vi "getClockInfo.vi"(8 "error in (no error)":errorcluster, 11 "DeviceData in":refnum<class "DeviceData.lvclass">) -> (0 "error out":errorcluster, 1 "masterClockRate":dbl, 2 "clock":string, 3 "DeviceData out":refnum<class "DeviceData.lvclass">, 4 "start_trigger":string)   [LabVIEW 2011, in "DataMappers.lvlib" / "DeviceData.lvclass"]
uses:
  DeviceData.lvclass
  DeviceData.lvclass/DeviceData.ctl
  DatabaseHelpers/Database Objects/device/device.lvclass
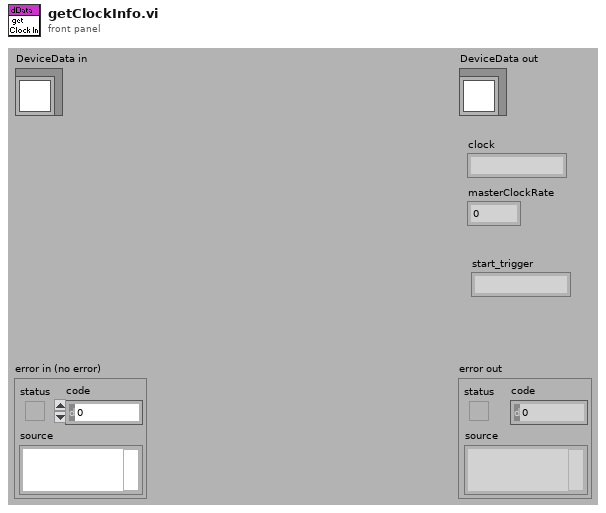
[diagram p1: front panel]
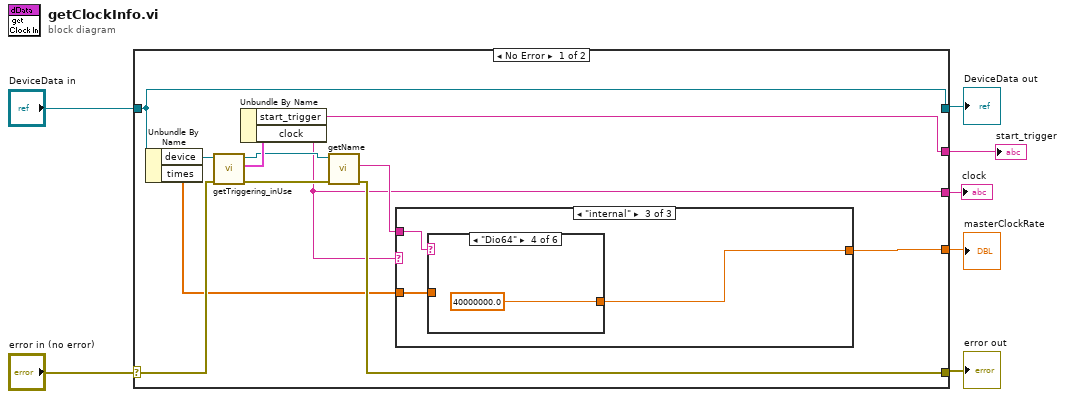
[diagram p0: block diagram]
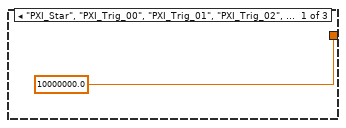
[diagram p2: hidden frame]
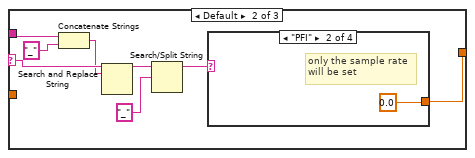
[diagram p3: hidden frame]
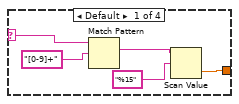
[diagram p4: hidden frame]
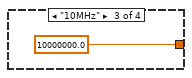
[diagram p5: hidden frame]
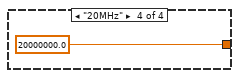
[diagram p6: hidden frame]
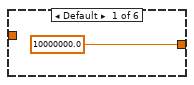
[diagram p7: hidden frame]
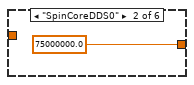
[diagram p8: hidden frame]
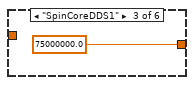
[diagram p9: hidden frame]
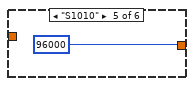
[diagram p10: hidden frame]
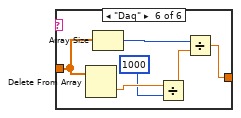
[diagram p11: hidden frame]
diagram:
  n1 = case shown="No Error" "error in (no error)" {
    selector: "error in (no error)" -> [w17 w52]
    tunnel: [w12 w52] -> w6
    tunnel: [w19 w51] -> w4
    tunnel: "DeviceData in" -> [w19 w51]
    tunnel: [w11 _] -> w3
    tunnel: [w10 _] -> w2
    tunnel: [w9 _] -> w1
    frame No Error {
      n2 = Unbundle By Name(w19) -> ("device"=w18:refnum<class "device.lvclass">, "times"=w8:dbl[])
      n3 = call "getTriggering_inUse.vi"("error in (no error)"=w17, "device.lvclass in"=w18) -> ("error out"=w14:errorcluster, "triggering_inUse"=w16:cluster{"start_trigger":string, "clock":string}, "device.lvclass out"=w15:refnum<class "device.lvclass">)  [unwired: 7 in]
      n4 = Unbundle By Name(w16) -> ("start_trigger"=w9:string, "clock"=w11:string)
      n5 = call "getName.vi"("error in (no error)"=w14, "device.lvclass in"=w15) -> ("error out"=w12:errorcluster, "name"=w13:string)  [unwired: 7 in, 1 out]
      n6 = case shown="\"internal\"" w11 {
        selector: w11 -> [_ w26 _]
        tunnel: w13 -> [_ w28 w39]
        tunnel: [10000000.0 w24 w38] -> w10
        tunnel: w8 -> [_ _ w37]
        frame "PXI_Star", "PXI_Trig_00", "PXI_Trig_01", "PXI_Trig_02", "PXI_Trig_03", "PXI_Trig_04", "PXI_Trig_05", "PXI_Trig_06", "PXI_Trig_07" {
        }
        frame Default {
          n7 = Concatenate Strings(w28, "_") -> (w25:string)
          n8 = Search and Replace String(input string=w26, search string=w25) -> (result string=w23:string)  [unwired: 6 in, 3 out]
          n9 = Search/Split String(string=w23, search string/char (-)="_") -> (substring before match=w21:string)  [unwired: 1 in, 2 out]
          n10 = case shown="\"PFI\"" w21 {
            selector: w21 -> [w33 _ _ _]
            tunnel: [w31 0.0 10000000.0 20000000.0] -> w24
            frame Default {
              n11 = Match Pattern(string=w33, regular expression="[0-9]+") -> (match substring=w30:string)  [unwired: 1 in, 3 out]
              n12 = Scan Value(string=w30, format string="%15") -> (value=w31:dbl)  [unwired: 1 in, 1 out]
            }
            frame "PFI" {
              # "only the sample rate\nwill be set"
            }
            frame "10MHz" {
            }
            frame "20MHz" {
            }
          }
        }
        frame "internal" {
          n13 = case shown="\"Dio64\"" w39 {
            tunnel: [10000000.0 75000000.0 75000000.0 40000000.0 96000 w45] -> w38
            tunnel: w37 -> [_ _ _ _ _ w50]
            frame Default {
            }
            frame "SpinCoreDDS0" {
            }
            frame "SpinCoreDDS1" {
            }
            frame "Dio64" {
            }
            frame "S1010" {
            }
            frame "Daq" {
              n14 = Delete From Array(array=w50) -> (deleted portion=w47:dbl)  [unwired: 2 in, 1 out]
              n15 = Array Size(array=w50) -> (size(s)=w49:i32)
              n16 = Divide(x=w47, y=1000) -> (x/y=w48:dbl)
              n17 = Divide(x=w49, y=w48) -> (x/y=w45:dbl)
            }
          }
        }
      }
    }
    frame Error {
    }
  }
  "error out" <- w6
  "DeviceData out" <- w4
  "clock" <- w3
  "masterClockRate" <- w2
  "start_trigger" <- w1
